vi "BCtr4.vi"() -> ()   [LabVIEW 2016]
uses:
  <vilib>/Platform/TimedLoop/XDataNode/timing_clust.ctl
  <vilib>/Platform/TimedLoop/XDataNode/nitl_modes.ctl
  <vilib>/Platform/TimedLoop/XDataNode/wakeup.ctl
  <vilib>/platform/TimedLoop/XDataNode/XDataNode.xnode
  <vilib>/Platform/TimedLoop/XDataNode/XDNodeRunTimeDep.lvlib
panel:
  out "Waveform Chart":u16(graph)
  out "LoopCt":dbl
  out "Ack":bool
  out "error out":errorcluster
  in  "Enable":bool
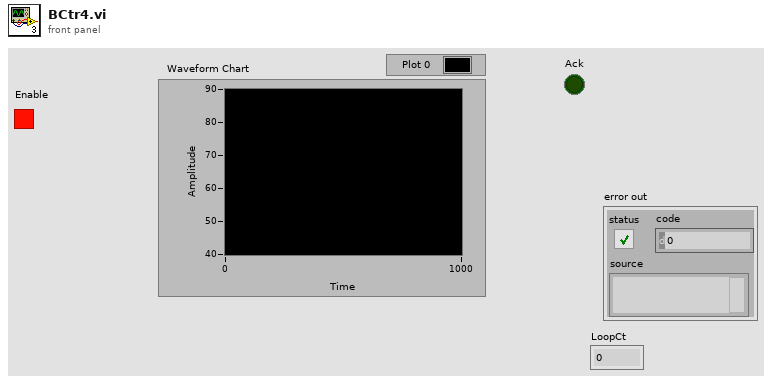
[diagram p1: front panel]
types:
  T1 = cluster{"Nbins":u16, "BaseAddrOut":u16, "PortOut":string, "ConfigOK":bool}
  T2 = typedef "XDNodeRunTimeDep.lvlib/timing_clust.ctl" = cluster{"Expected End [f-1]":u64, "Actual End [f-1]":u64, "Finished Late? [f-1]":bool, "Expected End [i-1]":u64, "Actual End [i-1]":u64, "Finished Late? [i-1]":bool, "Expected Start [i]":u64, "Actual Start [i]":u64, "Expected Start [f]":u64, "Actual Start [f]":u64, "Source Name":string, "Structure Name":string, "Period":i64, "Deadline":i64, "Offset":i64, "Start":i64, "Priority":i32, "Timeout":i32, "Mode":T3, "Wakeup Reason":T4, "Error":errorcluster, "Source Type":string, "Secondary Source Type":string, "Global End Time":u64, "Global Start Time":u64, "Frame Duration":u64, "Iteration Duration":u64, "Assigned CPU":i32, "I/O Scan Engine Mode":u32}
  T3 = typedef "XDNodeRunTimeDep.lvlib/nitl_modes.ctl" = enum32{"No Change", "Process missed periods, maintain original phase", "Discard missed periods, maintain original phase", "Process missed periods, ignore original phase", "Discard missed periods, ignore original phase"}
  T4 = typedef "XDNodeRunTimeDep.lvlib/wakeup.ctl" = enum32{"Normal", "Aborted", "Asynchronous wakeup", "Timing source error", "Timed loop error", "Timeout"}
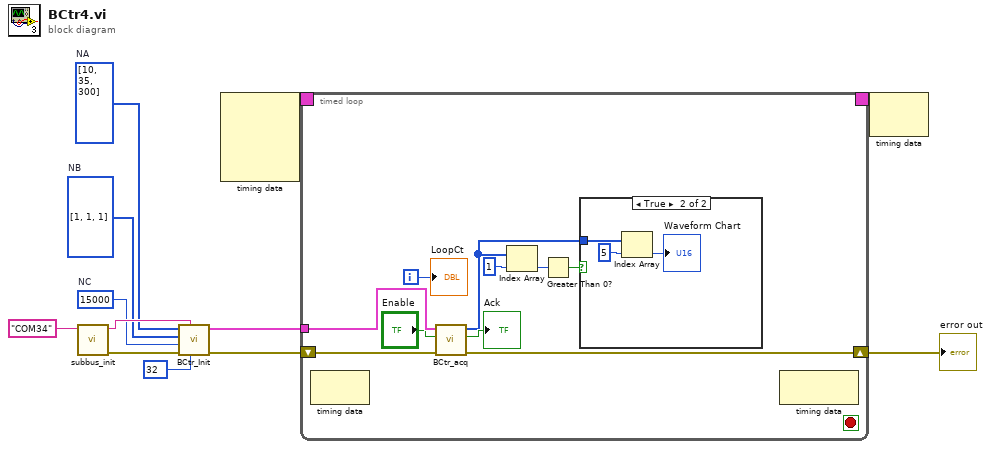
[diagram p0: block diagram]
diagram:
  w1 = 15000  # NC
  w2 = i32[] [1, 1, 1]  # NB
  w3 = i32[] [10, 35, 300]  # NA
  n1 = call "subbus_init.vi"("Port"="COM34") -> ("error out"=w11:errorcluster, "PortOut"=w12:string)  [unwired: 9 in]
  n2 = call "BCtr_Init.vi"("BaseAddr"=u16 32, "SBPort"=w12, "error in (no error)"=w11, "NC"=w1, "NB"=w2, "NA"=w3) -> ("error out"=w8:errorcluster, "CtrCfg"=w7:T1)  [unwired: 4 in]
  n3 = node-c288() -> (w5:T2)  [unwired: 4 in]
  n4 = timed-loop {
    timing: w5 -> [_]
    timing-out: [_] -> w4
    tunnel: w7 -> [w21]
    shift-right: [w20] -> w6
    shift-left: w8 -> [w22]
    i -> [w18]
    stop <- _ stop-if-true
    n5 = node-c288() -> ()  [unwired: 1 in, 1 out]
    n6 = call "BCtr_acq.vi"("error in (no error)"=w22, "Enable"="Enable", "CtrCfg"=w21) -> ("error out"=w20:errorcluster, "Ack"=→"Ack":bool, "Values"=w16:u16[])  [unwired: 6 in]
    n7 = Index Array(array=w16, index=1) -> (element=w14:u16)
    n8 = Greater Than 0?(x=w14) -> (x > 0?=w13:bool)
    n9 = case shown="True" w13 {
      tunnel: w16 -> [_ w25]
      frame False {
      }
      frame True {
        n10 = Index Array(array=w25, index=5) -> (element=→"Waveform Chart":u16)
      }
    }
    n11 = node-c288() -> ()  [unwired: 1 in, 1 out]
    "LoopCt" <- w18
  }
  "error out" <- w6
  n12 = node-c288(w4) -> ()  [unwired: 1 out]
